vi "Execute.vi"(8 "error in (no error)":errorcluster, 10 "Abstract Consumer in":refnum<class "Abstract Consumer.lvclass">, 11 "Log Message in":refnum<class "Check Size Message.lvclass">) -> (0 "error out":errorcluster, 1 "Abstract Response out":refnum<class "Abstract Response Message.lvclass">, 2 "Abstract Consumer out":refnum<class "Abstract Consumer.lvclass">, 3 "Log Message out":refnum<class "Check Size Message.lvclass">, 4 "Stop?":bool)   [LabVIEW 2020, in "AIM ARINC 664 Engine.lvlib" / "Implementation.lvlib" / "Frame Logging.lvlib" / "Check Size Message.lvclass"]
uses:
  Check Size Message.lvclass
  <vilib>/NI/VeriStand Custom Device Messaging/Consumer/Abstract Consumer/Abstract Consumer.lvclass
  <vilib>/NI/VeriStand Custom Device Messaging/Message/Abstract Response Message/Abstract Response Message.lvclass
  Check Size Message.lvclass/Check Size Message.ctl
  Read Logger.vi
  Read Log File Directory.vi
  Read Base name.vi
  Read Timestamp.vi
  Logger Interface/Logger Interface.lvclass
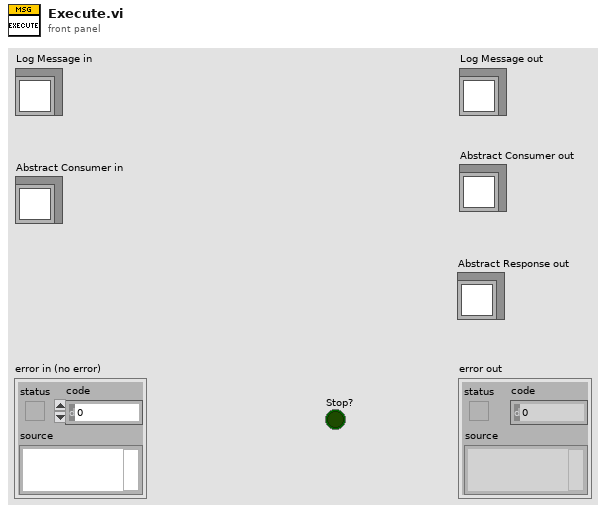
[diagram p1: front panel]
types:
  T1 = typedef "AIM ARINC 664 Engine.lvlib/Implementation.lvlib/Frame Logging.lvlib/Logger Data Reference.ctl" = refnum<data-value>
  T2 = cluster{"Logger Interface.lvclass":refnum<class "Logger Interface.lvclass">}
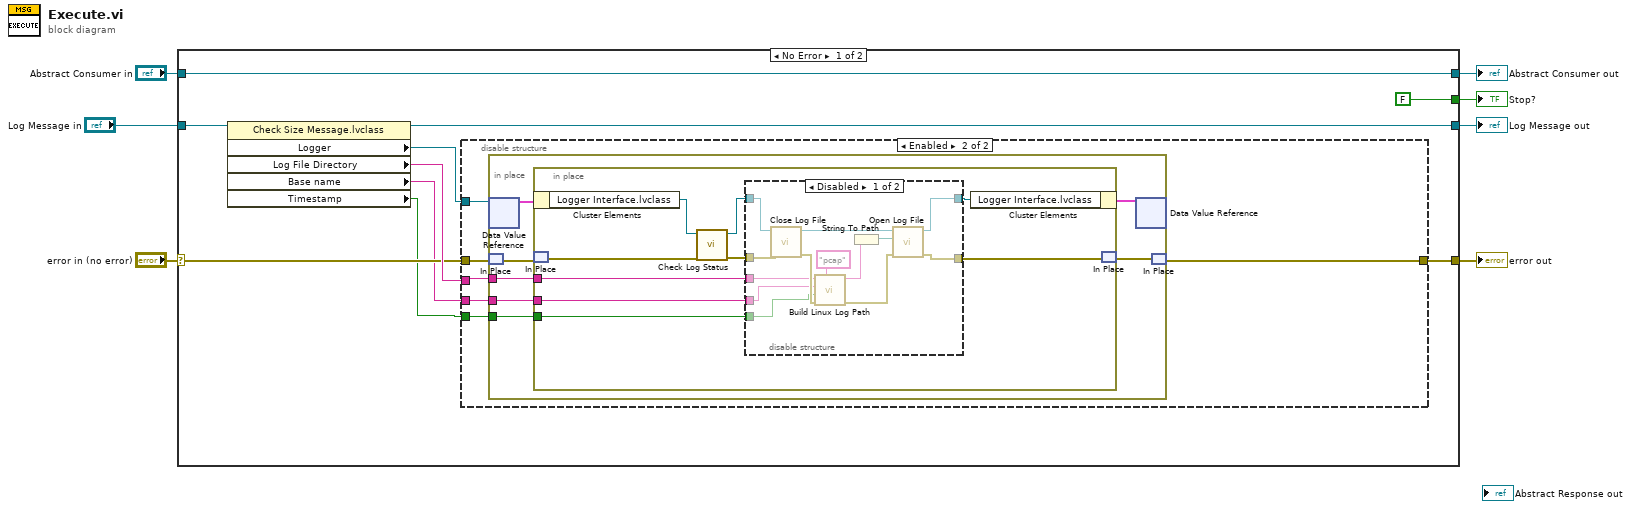
[diagram p0: block diagram]
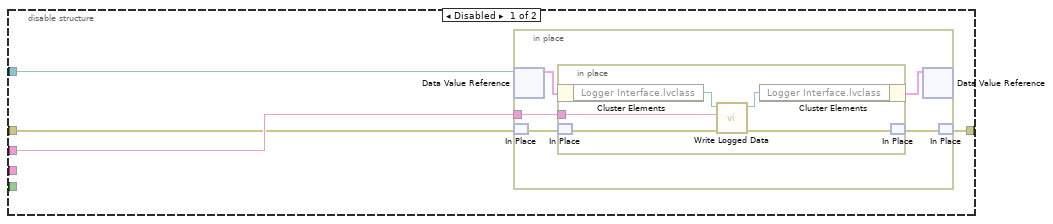
[diagram p2: hidden frame]
diagram:
  n1 = case shown="No Error" "error in (no error)" {
    selector: "error in (no error)" -> [w12 w71]
    tunnel: [w11 w71] -> w6
    tunnel: [w10 w70] -> w5
    tunnel: "Log Message in" -> [w15 w70]
    tunnel: [w16 w69] -> w3
    tunnel: "Abstract Consumer in" -> [w16 w69]
    tunnel: [FALSE ("Stop?") _] -> w1
    frame No Error {
      n2 = property class="Check Size Message.lvclass"(reference=w15) -> (reference out=w10:refnum<class "Check Size Message.lvclass">, "Logger"=w14:T1, "Log File Directory"=w13:string, "Base name"=w9:string, "Timestamp"=w8:bool)  [unwired: 1 in, 1 out]
      n3 = disable-structure shown="Enabled" {
        disable-tunnel: w14 -> [w21 w37]
        disable-tunnel: w13 -> [w20 w34]
        disable-tunnel: w12 -> [w19 w36]
        disable-tunnel: [w18 w35] -> w11
        disable-tunnel: w9 -> [_ w33]
        disable-tunnel: w8 -> [_ w32]
        frame Disabled {
          n4 = in-place {
            in-place-border: w20 -> [w25]
            n5 = in-place-dvr #1(w21) -> (w26:T2)  [unwired: 1 out]
            n6 = in-place-match #2(w19) -> (w24:errorcluster)
            n7 = in-place {
              in-place-border: w25 -> [w30]
              n8 = in-place-cluster #3(w26) -> ("Logger Interface.lvclass"=w31:refnum<class "Logger Interface.lvclass">)
              n9 = in-place-match #4(w24) -> (w29:errorcluster)
              n10 = call-dynamic "Write Logged Data.vi"("error in (no error)"=w29, "Data"=w30, "Logger Interface in"=w31) -> ("error out"=w28:errorcluster, "Logger Interface out"=w27:refnum<class "Logger Interface.lvclass">)  [unwired: 7 in]
              n11 = in-place-cluster #3("Logger Interface.lvclass"=w27) -> (w23:T2)
              n12 = in-place-match #4(w28) -> (w22:errorcluster)
            }
            n13 = in-place-dvr #1(w23) -> ()  [unwired: 2 out]
            n14 = in-place-match #2(w22) -> (w18:errorcluster)
          }
        }
        frame Enabled {
          n15 = in-place {
            in-place-border: w34 -> [w40]
            in-place-border: w33 -> [w39]
            in-place-border: w32 -> [w38]
            n16 = in-place-dvr #5(w37) -> (w44:T2)  [unwired: 1 out]
            n17 = in-place-match #6(w36) -> (w43:errorcluster)
            n18 = in-place {
              in-place-border: w40 -> [w47]
              in-place-border: w39 -> [w46]
              in-place-border: w38 -> [w45]
              n19 = in-place-cluster #7(w44) -> ("Logger Interface.lvclass"=w53:refnum<class "Logger Interface.lvclass">)
              n20 = in-place-match #8(w43) -> (w52:errorcluster)
              n21 = call-dynamic "Check Log Status.vi"("error in"=w52, "Logger Interface in"=w53) -> ("error out"=w49:errorcluster, "Logger Interface out"=w50:refnum<class "Logger Interface.lvclass">)  [unwired: 4 in, 4 out]
              n22 = disable-structure shown="Disabled" {
                disable-tunnel: [w62 w68] -> w51
                disable-tunnel: w50 -> [w66 w68]
                disable-tunnel: w49 -> [w64 w67]
                disable-tunnel: [w63 w67] -> w48
                disable-tunnel: w47 -> [w56 _]
                disable-tunnel: w46 -> [w55 _]
                disable-tunnel: w45 -> [w54 _]
                frame Disabled {
                  n23 = call-dynamic "Close Log File.vi"("error in (no error)"=w64, "Logger Interface in"=w66) -> ("error out"=w60:errorcluster, "Logger Interface out"=w65:refnum<class "Logger Interface.lvclass">)  [unwired: 8 in]
                  n24 = call "Build Linux Log Path.vi"("Extension"="pcap", "error in (no error)"=w60, "Timestamp"=w54, "Name"=w55, "Log File Directory"=w56) -> ("error out"=w59:errorcluster, "Log File Path"=w58:string)  [unwired: 5 in]
                  n25 = String To Path(string=w58) -> (path=w57:path)
                  n26 = call-dynamic "Open Log File.vi"("error in (no error)"=w59, "Path"=w57, "Logger Interface in"=w65) -> ("error out"=w63:errorcluster, "Logger Interface out"=w62:refnum<class "Logger Interface.lvclass">)  [unwired: 7 in]
                }
                frame Enabled {
                }
              }
              n27 = in-place-cluster #7("Logger Interface.lvclass"=w51) -> (w42:T2)
              n28 = in-place-match #8(w48) -> (w41:errorcluster)
            }
            n29 = in-place-dvr #5(w42) -> ()  [unwired: 2 out]
            n30 = in-place-match #6(w41) -> (w35:errorcluster)
          }
        }
      }
    }
    frame Error {
    }
  }
  "error out" <- w6
  "Log Message out" <- w5
  "Abstract Consumer out" <- w3
  "Stop?" <- w1
